vi "TTRM Analyze Temperature Measurements.vi"(0 "Temperature Waveforms In":waveform(dbl)[](array[waveform]), 11 "error in (no error)":errorcluster) -> (4 "Temperature Measurements Out":T1 {"Averaged Temperature (K)" format="%.2p"; "Averaged Temperature (degC)" format="%.2p"}, 15 "error out":errorcluster)   [LabVIEW 2021, in "DAQ_Temperature Thermistor Measurement.lvlib"]
doc: "Analyzes the temperature waveforms data obtained from analog input measurements to derive required temperature related measurements"
uses:
  DAQ_Temperature Thermistor Measurement.lvlib
  Typedefs/Temperature Thermistor Measurements.ctl
  <vilib>/Analysis/baseanly.llb/Mean (DBL).vi
  <vilib>/Analysis/NI_AALBase.lvlib
panel:
  # "Inputs"
  # "Outputs"
  # "Overview:\nThis VI does post processing on obtained temperature waveforms from analog input to give the required Temperature Measurements output\n\nInstructions:\n1. Input the captured temperature waveforms to the input controls\n2. Observe the analyzed temperature measurements output"
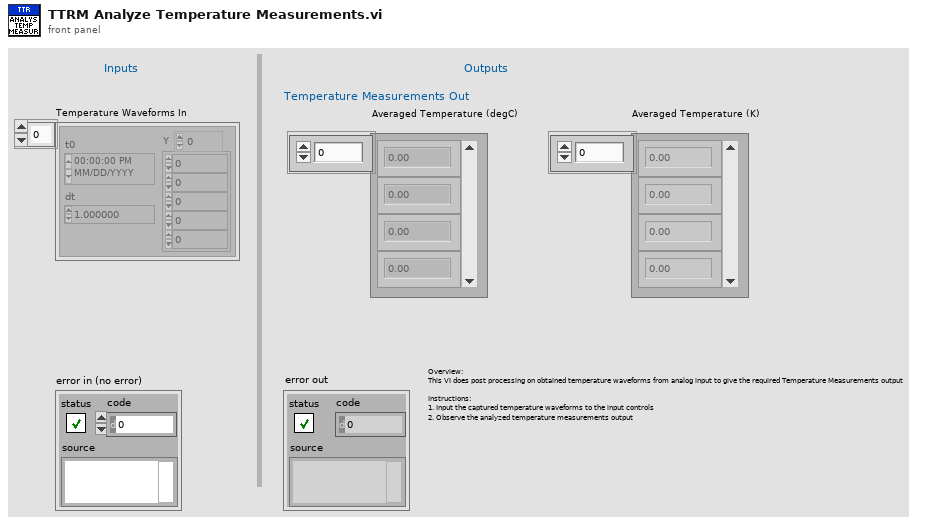
[diagram p1: front panel]
types:
  T1 = typedef "DAQ_Temperature Thermistor Measurement.lvlib/Temperature Thermistor Measurements.ctl" = cluster{"Averaged Temperature (degC)":dbl[], "Averaged Temperature (K)":dbl[]}
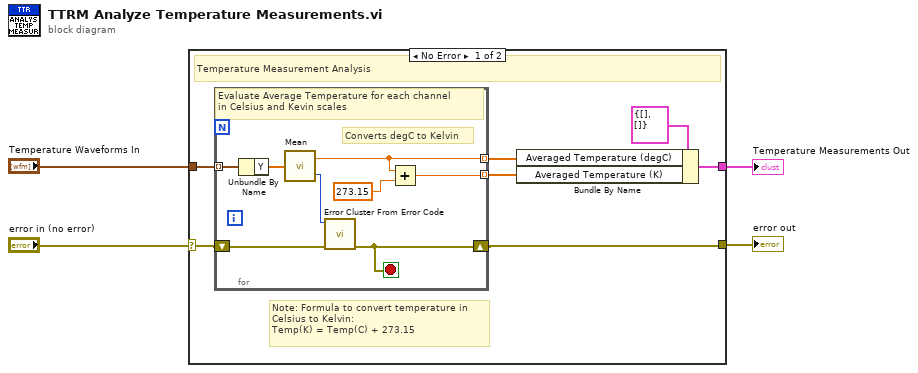
[diagram p0: block diagram]
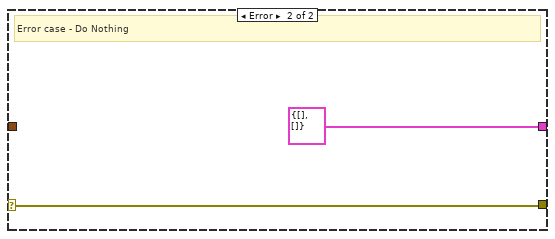
[diagram p2: hidden frame]
diagram:
  n1 = case shown="No Error" "error in (no error)" {
    selector: "error in (no error)" -> [w9 w21]
    tunnel: "Temperature Waveforms In" -> [w8 _]
    tunnel: [w10 T1 {"Averaged Temperature (degC)"=[], "Averaged Temperature (K)"=[]} ("Measure Settings")] -> w2
    tunnel: [w7 w21] -> w1
    frame No Error {
      # "Note: Formula to convert temperature in\nCelsius to Kelvin:\nTemp(K) = Temp(C) + 273.15"
      # "Temperature Measurement Analysis"
      n2 = for {
        shift-right: [w13] -> w7
        shift-left: w9 -> [w14]
        tunnel: w8 -> [w19] mode=indexing
        tunnel: [w16] -> w6 mode=indexing
        tunnel: [w15] -> w5 mode=indexing
        stop <- w13 stop-if-true
        # "Converts degC to Kelvin"
        # "Evaluate Average Temperature for each channel\nin Celsius and Kevin scales"
        n3 = Unbundle By Name(w19) -> ("Y"=w18:dbl[])
        n4 = call-poly <vilib>:"Mean.vi"("X"=w18) -> ("mean"=w16:dbl, "error"=w12:i32)
        n5 = call <vilib>:"Error Cluster From Error Code.vi"("error in (no error)"=w14, "error code (0)"=w12) -> ("error out"=w13:errorcluster)  [unwired: 7 in]
        n6 = Add(x=w16, y=273.15) -> (x+y=w15:dbl)
      }
      n7 = Bundle By Name(cluster=T1 {"Averaged Temperature (degC)"=[], "Averaged Temperature (K)"=[]} ("Measure Settings"), "Averaged Temperature (degC)"=w6, "Averaged Temperature (K)"=w5) -> (w10:T1)
    }
    frame Error {
      # "Error case - Do Nothing"
    }
  }
  "error out" <- w1
  "Temperature Measurements Out" <- w2
